vi "0 - ADC Test System Main.vi"() -> ()   [LabVIEW 2019]
uses:
  <vilib>/Utility/error.llb/DialogType.ctl
  <vilib>/VirtualBench/VirtualBench.lvlib
  <vilib>/DigilentWF/DigilentWF.lvlib
panel:
  in  "开始测试":bool caption="Start"
  out "DNL - Max":dbl format="%.2f"
  out "DNL - Min":dbl format="%.2f"
  out "INL - Min":dbl format="%.2f"
  out "INL - Max":dbl format="%.2f"
  out "SNR (dB)":dbl format="%.2f"
  out "SINAD (dB)":dbl format="%.2f"
  out "THD (dB)":dbl format="%.2f"
  out "测试进度":u8(slide) caption="Testing..." scale=0.0..100.0
  out "参数选项卡":T1(tab)
  out "Time Domain Graph":waveform(dbl)(graph)={"t0"=timestamp(0 s since 1904-01-01), "dt"=1e-05, "Y"=[]}
  out "Power Spectrum":cluster{"f0":dbl, "df":dbl, "magnitude":dbl[]}(graph)={"f0"=0.0, "df"=3.344369753519949, "magnitude"=[]}
  out "Fundamental Frequency":dbl=5000.052891743732 format="%.2p"
  out "THD Power Spectrum":cluster{"f0":dbl, "df":dbl, "magnitude":dbl[]}[](graph)
  out "SINAD Power Spectrum":cluster{"f0":dbl, "df":dbl, "magnitude":dbl[]}[](graph)
  out "SNR Power Spectrum":cluster{"f0":dbl, "df":dbl, "magnitude":dbl[]}[](graph)
  out "Differential Nonlinearity":cluster{i32, i32, "Y[i]=X[i]*a+b":dbl[]}(graph)={-127, 1, "Y[i]=X[i]*a+b"=[]}
  out "Integral Nonlinearity":cluster{dbl, i32, ext[]}(graph)={-127.5, 1, []}
  out "Transfer Curve":cluster{dbl[], i32[]}[](graph)
  in  "Trigger Type":T2(tab)=enum."Digital Trigger"
  in  "Digital Trigger Source":tag caption="Trigger Source (no change)"
  in  "Edge":i32(ring)=1 caption="Trigger Slope (no change)" items=["Rising", "Falling", "Either"]
  in  "Level (V)":dbl format="%0.2f"
  in  "Hysteresis (V)":dbl=0.17
  in  "Analog Trigger Source":tag="mso/1" caption="Trigger Source (no change)"
  in  "Slope":i32(ring) caption="Trigger Slope (no change)" items=["Rising", "Falling", "Either"]
  in  "Pattern Trigger Source":tag="mso/d0:7" caption="Trigger Source (no change)"
  in  "Trigger Pattern":string="1R0XX1X0" caption="Trigger Pattern (no change)"
  in  "Digital Channel(s)":tag caption="Channel"
  in  "PWS Channel":tag
  in  "Voltage Level (V)":dbl
  in  "Current Limit (A)":dbl
  in  "测试机台选择":tag
  # "基于IECUBE-3839的ADC自动化测试程序"
  # "硬件配置"
  # "DUT测试参数"
  # "设备选择"
  # "任务1：根据测试要求完成测试基台硬件配置"
  # "电源配置"
  # "逻辑分析仪配置"
  # "DUT测试结果"
  # "Triggers immediately after MSO Run VI executes."
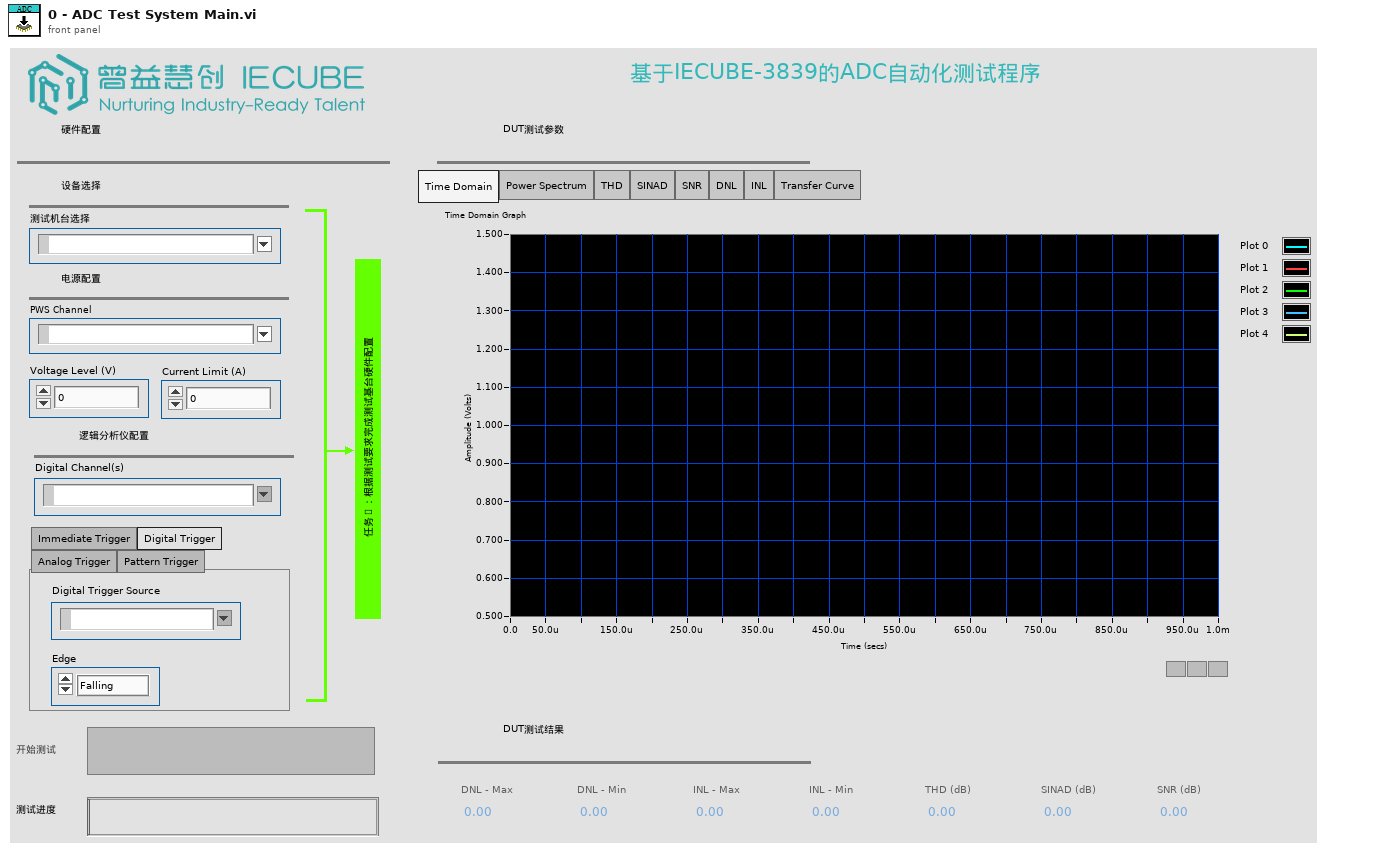
[diagram p1: front panel]
types:
  T1 = enum32{"Time Domain", "Power Spectrum", "THD", "SINAD", "SNR", "DNL", "INL", "Transfer Curve"}
  T2 = enum32{"Immediate Trigger", "Digital Trigger", "Analog Trigger", "Pattern Trigger"}
  T3 = enum8{"Enabled", "Disabled", "Disabled and Grayed Out"}
  T4 = cluster{"DNL - Max":refnum<vi>, "DNL - Min":refnum<vi>, "INL - Min":refnum<vi>, "INL - Max":refnum<vi>, "SNR (dB)":refnum<vi>, "SINAD (dB)":refnum<vi>, "THD (dB)":refnum<vi>, "测试进度":refnum<vi>, "参数选项卡":refnum<vi>, "Differential Nonlinearity":refnum<vi>, "Integral Nonlinearity":refnum<vi>, "Transfer Curve":refnum<vi>, "Time Domain Graph":refnum<vi>, "Fundamental Frequency":refnum<vi>, "THD Power Spectrum":refnum<vi>, "Power Spectrum":refnum<vi>, "SINAD Power Spectrum":refnum<vi>, "SNR Power Spectrum":refnum<vi>}
  T5 = cluster{"PWS Channel":tag, "Voltage Level (V)":dbl, "Current Limit (A)":dbl}
  T6 = cluster{"Trigger Type":enum32{"Immediate Trigger", "Digital Trigger", "Analog Trigger", "Pattern Trigger"}, "Digital Channel(s)":tag, "Analog Trigger Source":tag, "Slope":i32, "Level (V)":dbl, "Hysteresis (V)":dbl, "Digital Trigger Source":tag, "Edge":i32, "Pattern Trigger Source":tag, "Trigger Pattern":string}
  T7 = cluster{"DNL - Max":refnum<vi>, "DNL - Min":refnum<vi>, "INL - Min":refnum<vi>, "INL - Max":refnum<vi>, "SNR (dB)":refnum<vi>, "SINAD (dB)":refnum<vi>, "THD (dB)":refnum<vi>, "测试进度":refnum<vi>, "参数选项卡":refnum<vi>, "Differential Nonlinearity":refnum<vi>, "Integral Nonlinearity":refnum<vi>, "Transfer Curve":refnum<vi>, "Time Domain Graph":refnum<vi>, "Fundamental\nFrequency":refnum<vi>, "THD Power Spectrum":refnum<vi>, "Power Spectrum":refnum<vi>, "SINAD Power Spectrum":refnum<vi>, "SNR Power Spectrum":refnum<vi>}
  T8 = typedef "DialogType.ctl" = u16
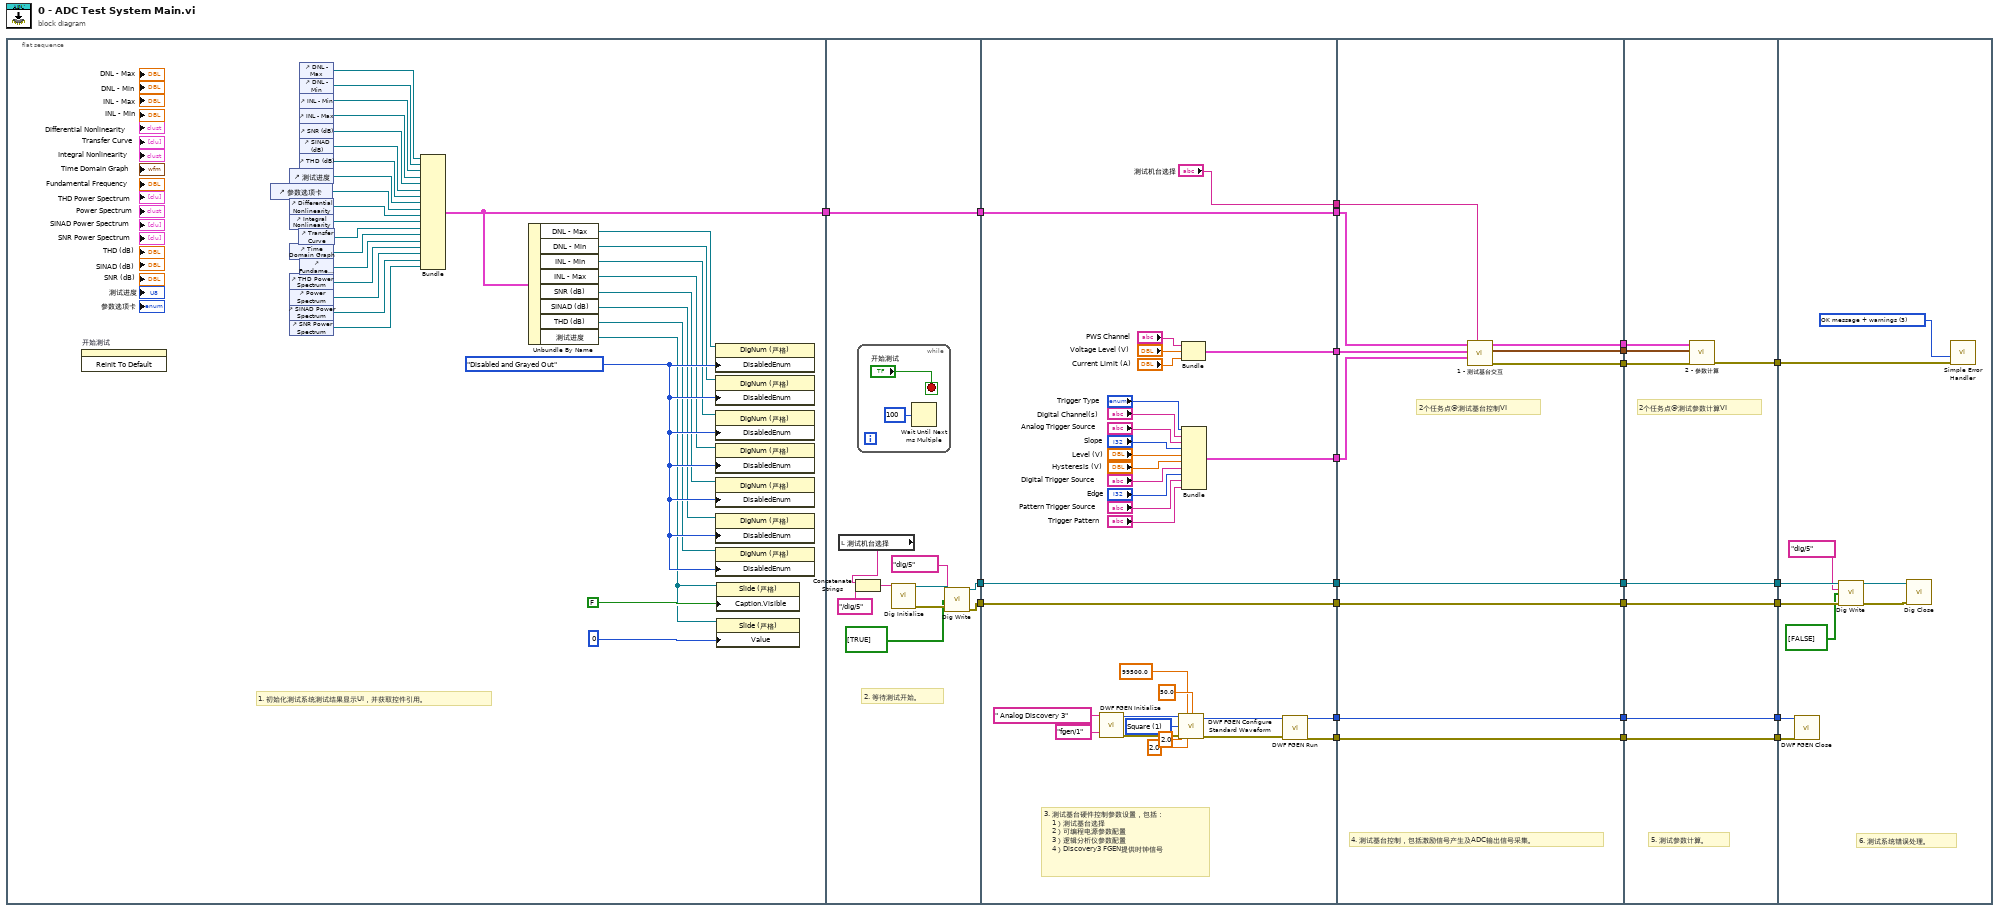
[diagram p0: block diagram]
diagram:
  n1 = flat-sequence {
    tunnel: [w25] -> w24
    tunnel: w24 -> [w64]
    tunnel: [w64] -> w23
    tunnel: [w58] -> w11
    tunnel: [w57] -> w7
    tunnel: w23 -> [w98]
    tunnel: [w98] -> w22
    tunnel: [w84] -> w21
    tunnel: [w83] -> w20
    tunnel: ["测试机台选择"] -> w19
    tunnel: [w81] -> w12
    tunnel: w11 -> [w81]
    tunnel: [w80] -> w8
    tunnel: w7 -> [w80]
    tunnel: [w68] -> w4
    tunnel: [w67] -> w3
    tunnel: w22 -> [w107]
    tunnel: w21 -> [w108]
    tunnel: w20 -> [w109]
    tunnel: w19 -> [w106]
    tunnel: [w105] -> w18
    tunnel: [w104] -> w17
    tunnel: [w103] -> w16
    tunnel: [w102] -> w13
    tunnel: w12 -> [w102]
    tunnel: [w101] -> w9
    tunnel: w8 -> [w101]
    tunnel: [w100] -> w5
    tunnel: w4 -> [w100]
    tunnel: w3 -> [w99]
    tunnel: [w99] -> w2
    tunnel: w18 -> [w117]
    tunnel: w17 -> [w116]
    tunnel: w16 -> [w115]
    tunnel: [w114] -> w15
    tunnel: [w113] -> w14
    tunnel: w13 -> [w113]
    tunnel: [w112] -> w10
    tunnel: w9 -> [w112]
    tunnel: [w111] -> w6
    tunnel: w5 -> [w111]
    tunnel: w2 -> [w110]
    tunnel: [w110] -> w1
    tunnel: w15 -> [w126]
    tunnel: w14 -> [w125]
    tunnel: w10 -> [w124]
    tunnel: w6 -> [w119]
    tunnel: w1 -> [w118]
    frame #0 {
      w36 = T3."Disabled and Grayed Out" ("禁用")
      # "1. 初始化测试系统测试结果显示UI，并获取控件引用。"
      n2 = invoke on="开始测试" class="Bool (严格)" method="Reinit To Default"() -> ()  [unwired: 3 in, 3 out]
      n3 = control-ref of="参数选项卡"() -> (w46:refnum<vi>)
      n4 = control-ref of="测试进度"() -> (w47:refnum<vi>)
      n5 = control-ref of="Differential Nonlinearity"() -> (w45:refnum<vi>)
      n6 = control-ref of="Integral Nonlinearity"() -> (w44:refnum<vi>)
      n7 = control-ref of="Time Domain Graph"() -> (w42:refnum<vi>)
      n8 = control-ref of="THD Power Spectrum"() -> (w40:refnum<vi>)
      n9 = control-ref of="Power Spectrum"() -> (w39:refnum<vi>)
      n10 = control-ref of="SINAD Power Spectrum"() -> (w38:refnum<vi>)
      n11 = control-ref of="SNR Power Spectrum"() -> (w37:refnum<vi>)
      n12 = control-ref of="Transfer Curve"() -> (w43:refnum<vi>)
      n13 = control-ref of="DNL - Max"() -> (w54:refnum<vi>)
      n14 = control-ref of="DNL - Min"() -> (w53:refnum<vi>)
      n15 = control-ref of="INL - Min"() -> (w52:refnum<vi>)
      n16 = control-ref of="INL - Max"() -> (w51:refnum<vi>)
      n17 = control-ref of="SNR (dB)"() -> (w50:refnum<vi>)
      n18 = control-ref of="SINAD (dB)"() -> (w49:refnum<vi>)
      n19 = control-ref of="THD (dB)"() -> (w48:refnum<vi>)
      n20 = control-ref of="Fundamental Frequency"() -> (w41:refnum<vi>)
      n21 = Bundle("DNL - Max"=w54, "DNL - Min"=w53, "INL - Min"=w52, "INL - Max"=w51, "SNR (dB)"=w50, "SINAD (dB)"=w49, "THD (dB)"=w48, "测试进度"=w47, "参数选项卡"=w46, "Differential Nonlinearity"=w45, "Integral Nonlinearity"=w44, "Transfer Curve"=w43, "Time Domain Graph"=w42, "Fundamental Frequency"=w41, "THD Power Spectrum"=w40, "Power Spectrum"=w39, "SINAD Power Spectrum"=w38, "SNR Power Spectrum"=w37) -> (w25:T4)  [unwired: 1 in]
      n22 = Unbundle By Name(w25) -> ("DNL - Max"=w33:refnum<vi>, "DNL - Min"=w32:refnum<vi>, "INL - Min"=w31:refnum<vi>, "INL - Max"=w30:refnum<vi>, "SNR (dB)"=w29:refnum<vi>, "SINAD (dB)"=w28:refnum<vi>, "THD (dB)"=w27:refnum<vi>, "测试进度"=w26:refnum<vi>)
      n23 = property class="DigNum (严格)"(reference=w33, "DisabledEnum"=w36) -> ()  [unwired: 1 in, 2 out]
      n24 = property class="DigNum (严格)"(reference=w32, "DisabledEnum"=w36) -> ()  [unwired: 1 in, 2 out]
      n25 = property class="DigNum (严格)"(reference=w31, "DisabledEnum"=w36) -> ()  [unwired: 1 in, 2 out]
      n26 = property class="DigNum (严格)"(reference=w30, "DisabledEnum"=w36) -> ()  [unwired: 1 in, 2 out]
      n27 = property class="DigNum (严格)"(reference=w29, "DisabledEnum"=w36) -> ()  [unwired: 1 in, 2 out]
      n28 = property class="DigNum (严格)"(reference=w28, "DisabledEnum"=w36) -> ()  [unwired: 1 in, 2 out]
      n29 = property class="DigNum (严格)"(reference=w27, "DisabledEnum"=w36) -> ()  [unwired: 1 in, 2 out]
      n30 = property class="Slide (严格)"(reference=w26, "Caption.Visible"=FALSE ("标题.可见")) -> ()  [unwired: 1 in, 2 out]
      n31 = property class="Slide (严格)"(reference=w26, "Value"=u8 0 ("值")) -> ()  [unwired: 1 in, 2 out]
    }
    frame #1 {
      # "2. 等待测试开始。"
      n32 = local read "测试机台选择"() -> (w61:tag)
      n33 = Concatenate Strings(w61, "/dig/5" ("字符串")) -> (w60:string)
      n34 = while {
        stop <- "开始测试" stop-if-true
        n35 = Wait Until Next ms Multiple(millisecond multiple=u32 100) -> ()  [unwired: 1 out]
      }
      n36 = call <vilib>:"Dig Initialize.vi"("Lines"=w60) -> ("Instrument Handle Out"=w63:refnum<k21>, "Error Out"=w62:errorcluster)  [unwired: 13 in]
      n37 = call <vilib>:"Dig Write.vi"("Instrument Handle In"=w63, "Lines"=tag "dig/5", "Data"=bool[] [TRUE], "Error In"=w62) -> ("Instrument Handle Out"=w58:refnum<k21>, "Error Out"=w57:errorcluster)  [unwired: 10 in]
    }
    frame #2 {
      w73 = 1 items=["Sine", "Square", "Triangle/Ramp", "DC"] ("Waveform Function")
      # "3. 测试基台硬件控制参数设置，包括：\n    1）测试基台选择\n    2）可编程电源参数配置\n    3）逻辑分析仪参数配置\n    4）Discovery3 FGEN提供时钟信号"
      n38 = call <vilib>:"DWF FGEN Initialize.vi"("Device Name"=" Analog Discovery 3", "Channel"="fgen/1") -> ("Instrument Handle Out"=w74:u32, "Error Out"=w77:errorcluster)  [unwired: 12 in]
      n39 = call <vilib>:"DWF FGEN Configure Standard Waveform.vi"("Instrument Handle In"=w74, "Frequency"=99500.0, "Duty Cycle"=50.0, "Waveform Function"=w73, "Amplitude"=2.0, "Error In"=w77, "DC Offset"=2.0) -> ("Instrument Handle Out"=w75:u32, "Error Out"=w76:errorcluster)  [unwired: 7 in]
      n40 = Bundle("PWS Channel"="PWS Channel", "Voltage Level (V)"="Voltage Level (V)", "Current Limit (A)"="Current Limit (A)") -> (w83:T5)  [unwired: 1 in]
      n41 = Bundle("Trigger Type"="Trigger Type", "Digital Channel(s)"="Digital Channel(s)", "Analog Trigger Source"="Analog Trigger Source", "Slope"="Slope", "Level (V)"="Level (V)", "Hysteresis (V)"="Hysteresis (V)", "Digital Trigger Source"="Digital Trigger Source", "Edge"="Edge", "Pattern Trigger Source"="Pattern Trigger Source", "Trigger Pattern"="Trigger Pattern") -> (w84:T6)  [unwired: 1 in]
      n42 = call <vilib>:"DWF FGEN Run.vi"("Instrument Handle In"=w75, "Error In"=w76) -> ("Instrument Handle Out"=w68:u32, "Error Out"=w67:errorcluster)  [unwired: 12 in]
    }
    frame #3 {
      # "2个任务点@测试基台控制VI"
      # "4. 测试基台控制，包括激励信号产生及ADC输出信号采集。"
      n43 = call "1 - 测试基台交互.vi"("测试机台选择"=w106, "逻辑分析仪参数输入"=w108, "可编程电源参数输入"=w109, "显示控件引用输入"=w107) -> ("error out"=w103:errorcluster, "采集信号输出"=w104:waveform(dbl)[], "显示控件引用输出"=w105:T7)  [unwired: 4 in]
    }
    frame #4 {
      # "2个任务点@测试参数计算VI"
      # "5. 测试参数计算。"
      n44 = call "2 - 参数计算.vi"("error in (no error)"=w115, "采集信号输入"=w116, "显示控件引用输入"=w117) -> ("error out"=w114:errorcluster)  [unwired: 8 in]
    }
    frame #5 {
      w127 = T8 3 items=["no dialog", "OK message", "continue or stop message", "OK message + warnings", "continue/stop + warnings"] ("type of dialog (OK msg:1)")
      # "6. 测试系统错误处理。"
      n45 = call <vilib>:"DWF FGEN Close.vi"("Instrument Handle In"=w119, "Error In"=w118) -> ()  [unwired: 13 in, 1 out]
      n46 = call <vilib>:"Dig Write.vi"("Instrument Handle In"=w125, "Lines"=tag "dig/5", "Data"=bool[] [FALSE], "Error In"=w124) -> ("Instrument Handle Out"=w123:refnum<k21>, "Error Out"=w122:errorcluster)  [unwired: 10 in]
      n47 = call <vilib>:"Dig Close.vi"("Instrument Handle In"=w123, "Error In"=w122) -> ()  [unwired: 13 in, 1 out]
      n48 = call <vilib>:"Simple Error Handler.vi"("type of dialog (OK msg:1)"=w127, "error in (no error)"=w126) -> ()  [unwired: 3 in, 5 out]
    }
  }
